vi "UI_Elmt_Read_MAP.vi"(8 "error in (no error)":errorcluster, 11 "UI_Actor in":refnum<class "UI_Actor.lvclass">) -> (0 "error out":errorcluster, 2 "UI Refs Map":map{string, refnum<vi>}(c390), 3 "UI_Actor out":refnum<class "UI_Actor.lvclass">)   [LabVIEW 2020, in "UI_Actor.lvlib" / "UI_Actor.lvclass"]
doc: "Accès à un élément par son label.\n<b> NEVER USE IN FOR LOOP </b> \nLa ref est stockée au premier appel en fgv.\nLe VI doit etre dédié à un unique élement."
uses:
  UI_Actor.lvclass
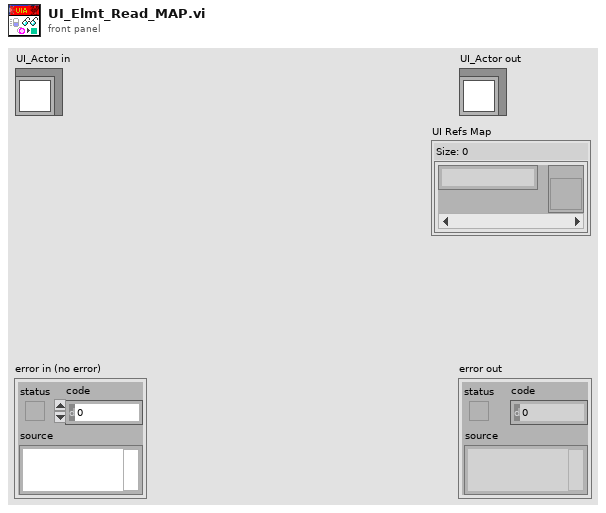
[diagram p1: front panel]
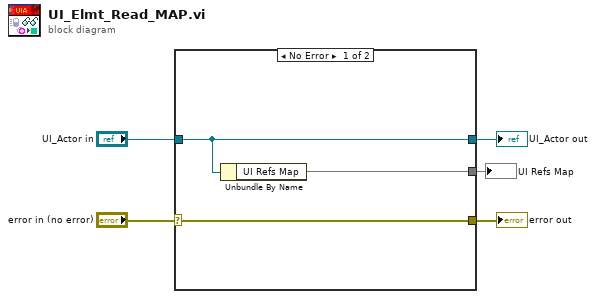
[diagram p0: block diagram]
diagram:
  n1 = case shown="No Error" "error in (no error)" {
    selector: "error in (no error)" -> [w7 w10]
    tunnel: [w7 w10] -> w4
    tunnel: [w8 w9] -> w2
    tunnel: "UI_Actor in" -> [w8 w9]
    tunnel: [w6 _] -> w1
    frame No Error {
      n2 = Unbundle By Name(w8) -> ("UI Refs Map"=w6:map{string, refnum<vi>})
    }
    frame Error {
    }
  }
  "error out" <- w4
  "UI_Actor out" <- w2
  "UI Refs Map" <- w1
